vi "Read Params.vi"(8 "error in (no error)":errorcluster, 11 "KD Tree in":refnum<class "KD Tree.lvclass">) -> (0 "error out":errorcluster, 2 "data value":T1={"algorithm"=0, "checks"=0, "eps"=0.0, "sorted"=1, "max_neighbors"=-1, "cores"=0, "trees"=0, "leaf_max_size"=0, "branching"=0, "iterations"=0, "centers_init"=0, "cb_index"=0.0, "target_precision"=0.0, "build_weight"=0.0, "memory_weight"=0.0, "sample_fraction"=0.0, "table_number_"=0, "key_size_"=0, "multi_probe_level_"=0, "log_level"=0, "random_seed"=0} {"algorithm" items=["FLANN_INDEX_LINEAR"=0, "FLANN_INDEX_KDTREE"=1, "FLANN_INDEX_KMEANS"=2, "FLANN_INDEX_COMPOSITE"=3, "FLANN_INDEX_KDTREE_SINGLE"=4, "FLANN_INDEX_HIERARCHICAL"=5, "FLANN_INDEX_LSH"=6, "FLANN_INDEX_SAVED"=254, "FLANN_INDEX_AUTOTUNED"=255]; "centers_init" items=["FLANN_CENTERS_RANDOM", "FLANN_CENTERS_GONZALES", "FLANN_CENTERS_KMEANSPP", "FLANN_CENTERS_GROUPWISE"]; "log_level" items=["FLANN_LOG_NONE", "FLANN_LOG_FATAL", "FLANN_LOG_ERROR", "FLANN_LOG_WARN", "FLANN_LOG_INFO", "FLANN_LOG_DEBUG"]}, 3 "KD Tree out":refnum<class "KD Tree.lvclass">)   [LabVIEW 2020, in "KD Tree.lvlib" / "KD Tree.lvclass"]
uses:
  KD Tree.lvclass
  flann/Flann Params.ctl
  KD Tree.lvlib
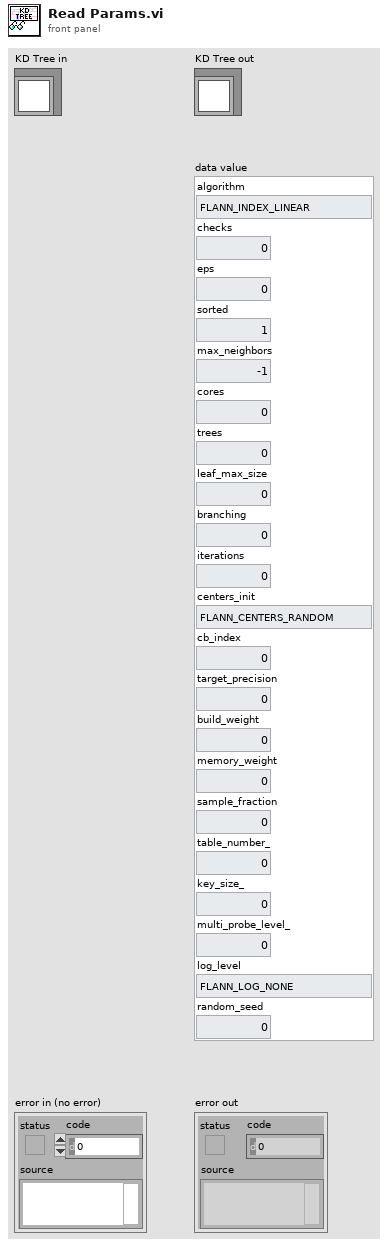
[diagram p1: front panel]
types:
  T1 = typedef "KD Tree.lvlib/Flann Params.ctl" = cluster{"algorithm":u32, "checks":i32, "eps":sgl, "sorted":i32, "max_neighbors":i32, "cores":i32, "trees":i32, "leaf_max_size":i32, "branching":i32, "iterations":i32, "centers_init":u32, "cb_index":sgl, "target_precision":sgl, "build_weight":sgl, "memory_weight":sgl, "sample_fraction":sgl, "table_number_":u32, "key_size_":u32, "multi_probe_level_":u32, "log_level":u32, "random_seed":i32}
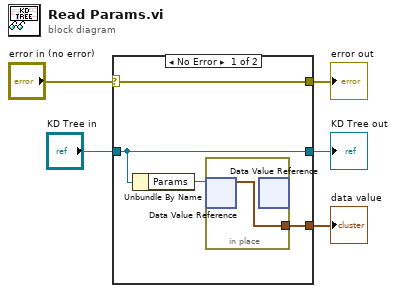
[diagram p0: block diagram]
diagram:
  n1 = case shown="No Error" "error in (no error)" {
    selector: "error in (no error)" -> [w9 w11]
    tunnel: [w9 w11] -> w4
    tunnel: [w8 w12] -> w2
    tunnel: "KD Tree in" -> [w8 w12]
    tunnel: [w6 _] -> w1
    frame No Error {
      n2 = Unbundle By Name(w8) -> ("Params"=w7:refnum<data-value>)
      n3 = in-place {
        in-place-border: [w10] -> w6
        n4 = in-place-dvr #1(w7) -> (w10:T1)  [unwired: 1 out]
        n5 = in-place-dvr #1() -> ()  [unwired: 1 in, 2 out]
      }
    }
    frame Error {
    }
  }
  "error out" <- w4
  "KD Tree out" <- w2
  "data value" <- w1
